vi "Counter - Continuous Output-no trigger.vi"() -> ()   [LabVIEW 2014]
doc: "This example demonstrates how to continuously generate digital pulses using a counter output."
uses:
  <vilib>/Utility/error.llb/DialogType.ctl
  <vilib>/DAQmx/create/channels.llb/DAQmx Create Channel (CO-Pulse Generation-Frequency).vi
  <vilib>/DAQmx/create/channels.llb/DAQmx Create Channel (CO-Pulse Generation-Time).vi
  <vilib>/DAQmx/configure/timing.llb/DAQmx Timing (Implicit).vi
  <resource>/objmgr/daqmx.rc
panel:
  in  "Mode":enum32{"Frequency", "Time"}(tab)
  in  "Frequency":dbl=1.0 format="%.6f"
  in  "Duty Cycle":dbl=0.5 format="%.6f"
  out "Actual Frequency":dbl
  out "Actual Duty Cycle":dbl
  out "Actual High Time":dbl
  out "Actual Low Time":dbl
  in  "Low Time":dbl=0.5 format="%.6f"
  in  "High Time":dbl=1.0 format="%.6f"
  in  "Output Terminal":tag="/Dev1/PFI12"
  in  "Stop":bool
  in  "Counter":tag="Dev1/ctr0"
  # "Channel Settings"
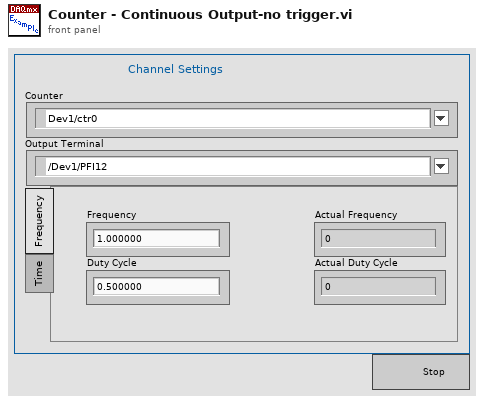
[diagram p1: front panel]
types:
  T1 = typedef "DialogType.ctl" = u16
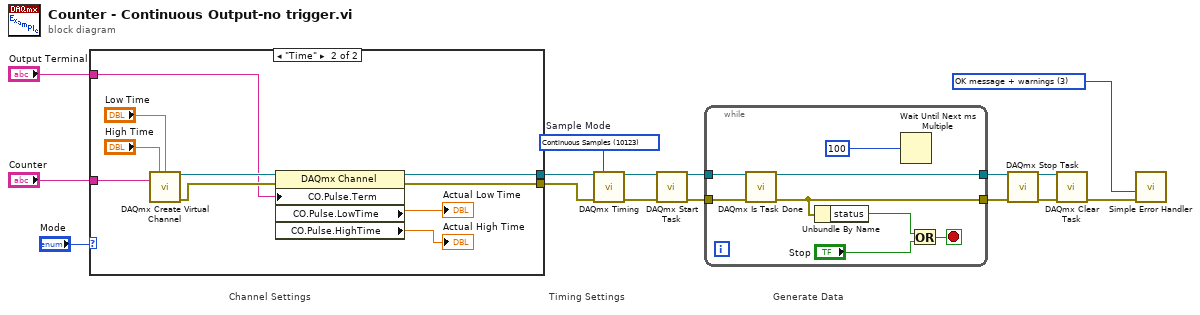
[diagram p0: block diagram]
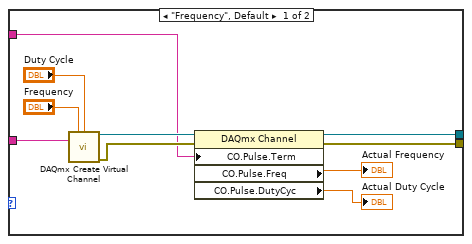
[diagram p2: hidden frame]
diagram:
  w5 = T1 3 items=["no dialog", "OK message", "continue or stop message", "OK message + warnings", "continue/stop + warnings"] ("type of dialog (OK msg:1)")
  w16 = 10123 items=["Finite Samples"=10178, "Continuous Samples"=10123, "Hardware Timed Single Point"=12522]  # Sample Mode
  # "Generate Data"
  # "Timing Settings"
  # "Channel Settings"
  n1 = case shown="\"Time\"" "Mode" {
    tunnel: "Counter" -> [w26 w36]
    tunnel: "Output Terminal" -> [w23 w33]
    tunnel: [w22 w32] -> w10
    tunnel: [w17 w27] -> w2
    frame "Frequency", Default {
      n2 = call-poly <vilib>:"DAQmx Create Virtual Channel.vi"("frequency"="Frequency", "duty cycle"="Duty Cycle", "counter"=w26) -> ("task out"=w25:refnum<k21>, "error out"=w24:errorcluster)  [unwired: 11 in]
      n3 = property class="DAQmx Channel"(reference=w25, error in=w24, "CO.Pulse.Term"=w23) -> (reference out=w22:refnum<k21>, error out=w17:errorcluster, "CO.Pulse.Freq"=→"Actual Frequency":dbl, "CO.Pulse.DutyCyc"=→"Actual Duty Cycle":dbl)
    }
    frame "Time" {
      n4 = call-poly <vilib>:"DAQmx Create Virtual Channel.vi"("high time"="High Time", "low time"="Low Time", "counter"=w36) -> ("task out"=w35:refnum<k21>, "error out"=w34:errorcluster)  [unwired: 11 in]
      n5 = property class="DAQmx Channel"(reference=w35, error in=w34, "CO.Pulse.Term"=w33) -> (reference out=w32:refnum<k21>, error out=w27:errorcluster, "CO.Pulse.LowTime"=→"Actual Low Time":dbl, "CO.Pulse.HighTime"=→"Actual High Time":dbl)
    }
  }
  n6 = call-poly <vilib>:"DAQmx Timing.vi"("task/channels in"=w10, "sample mode"=w16, "error in"=w2) -> ("task out"=w4:refnum<k21>, "error out"=w3:errorcluster)  [unwired: 11 in]
  n7 = call <vilib>:"DAQmx Start Task.vi"("task/channels in"=w4, "error in"=w3) -> ("task out"=w15:refnum<k21>, "error out"=w14:errorcluster)  [unwired: 12 in]
  n8 = while {
    tunnel: w15 -> [w44]
    tunnel: w14 -> [w43]
    tunnel: [w40] -> w6
    tunnel: [w41] -> w7
    stop <- w42 stop-if-true
    n9 = call <vilib>:"DAQmx Is Task Done.vi"("task/channels in"=w44, "error in"=w43) -> ("task out"=w41:refnum<k21>, "error out"=w40:errorcluster)  [unwired: 11 in, 1 out]
    n10 = Unbundle By Name(w40) -> ("status"=w39:bool)
    n11 = Wait Until Next ms Multiple(millisecond multiple=u32 100) -> ()  [unwired: 1 out]
    n12 = Or(x=w39, y="Stop") -> (x .or. y?=w42:bool)
  }
  n13 = call <vilib>:"DAQmx Stop Task.vi"("task/channels in"=w7, "error in"=w6) -> ("task out"=w9:refnum<k21>, "error out"=w8:errorcluster)  [unwired: 12 in]
  n14 = call <vilib>:"DAQmx Clear Task.vi"("task in"=w9, "error in"=w8) -> ("error out"=w13:errorcluster)  [unwired: 13 in]
  n15 = call <vilib>:"Simple Error Handler.vi"("type of dialog (OK msg:1)"=w5, "error in (no error)"=w13) -> ()  [unwired: 3 in, 5 out]
